vi "spl.vi"() -> ()   [LabVIEW 2017]
doc: "Performs limit testing on unevenly sampled data. You might have unevenly sampled data in some applications, such as data sampled on a logarithmic scale.\n\nThis example uses the Limit Specification for Unevenly Sampled Data subVI. If you do not wire the dx and the x0 inputs, this VI accepts an array of X axis values at which your signal is sampled. It creates the limit at these X values. The example then uses the Limit Testing VI to compare the signal with the limits."
uses:
  <vilib>/measure/mamon.llb/Limit Testing Time.vi
  <vilib>/measure/NI_MAPro.lvlib
panel:
  in  "声压级":dbl[](array[numeric])=[82.29, 84.67, 86.31, 87.22, 86.54, 84.99, 83.09, 82.19, 82.2, 83.13, 84.47, 86.53, 88.83, 91.58, 93.49, 94.45, 94.45, 93.83, 93.46, 94.46, 97.18, 99.83, 101.28, 102.07, 102.67, 103.01, 102.91, 102.6, 101.82, 100.98, 99.07, 98.85, 101.46, 101.31, 99.62, 101.88, 104.09, 102.62, 103.66, 103.86, 104.63, 105.12, 105.52, 103.79, 103.37, 103.81, 105.35, 105.82, 105.16, 103.88, 102.23, 101.82, 102.49, 102.97, 100.5, 101.51, 101.54, 101.41, 101.61, 101.8, 102.8]
  in  "频率":dbl[](array[numeric])=[204.0, 216.0, 227.0, 241.0, 255.0, 270.0, 285.0, 302.0, 319.0, 338.0, 357.0, 378.0, 399.0, 422.0, 446.0, 472.0, 499.0, 528.0, 558.0, 590.0, 623.0, 659.0, 697.0, 736.0, 778.0, 823.0, 870.0, 919.0, 972.0, 1025.0, 1086.0, 1149.0, 1214.0, 1288.0, 1358.0, 1435.0, 1517.0, 1606.0, 1695.0, 1796.0, 1898.0, 2005.0, 2130.0, 2242.0, 2371.0, 2508.0, 2649.0, 2802.0, 2961.0, 3126.0, 3315.0, 3500.0, 3695.0, 3911.0, 4136.0, 4372.0, 4630.0, 4889.0, 5169.0, 5461.0, 5783.0]
  out "test passed?":bool=TRUE
  out "Limit Test":T1(graph)=[{"X Values for Signal"=[204.0, 216.0, 227.0, 241.0, 255.0, 270.0, 285.0, 302.0, 319.0, 338.0, 357.0, 378.0, 399.0, 422.0, 446.0, 472.0, 499.0, 528.0, 558.0, 590.0, 623.0, 659.0, 697.0, 736.0, 778.0, 823.0, 870.0, 919.0, 972.0, 1025.0, 1086.0, 1149.0, 1214.0, 1288.0, 1358.0, 1435.0, 1517.0, 1606.0, 1695.0, 1796.0, 1898.0, 2005.0, 2130.0, 2242.0, 2371.0, 2508.0, 2649.0, 2802.0, 2961.0, 3126.0, 3315.0, 3500.0, 3695.0, 3911.0, 4136.0, 4372.0, 4630.0, 4889.0, 5169.0, 5461.0, 5783.0], "Y"=[82.29, 84.67, 86.31, 87.22, 86.54, 84.99, 83.09, 82.19, 82.2, 83.13, 84.47, 86.53, 88.83, 91.58, 93.49, 94.45, 94.45, 93.83, 93.46, 94.46, 97.18, 99.83, 101.28, 102.07, 102.67, 103.01, 102.91, 102.6, 101.82, 100.98, 99.07, 98.85, 101.46, 101.31, 99.62, 101.88, 104.09, 102.62, 103.66, 103.86, 104.63, 105.12, 105.52, 103.79, 103.37, 103.81, 105.35, 105.82, 105.16, 103.88, 102.23, 101.82, 102.49, 102.97, 100.5, 101.51, 101.54, 101.41, 101.61, 101.8, 102.8]}, {"X Values for Signal"=[204.0, 216.0, 227.0, 241.0, 255.0, 270.0, 285.0, 302.0, 319.0, 338.0, 357.0, 378.0, 399.0, 422.0, 446.0, 472.0, 499.0, 528.0, 558.0, 590.0, 623.0, 659.0, 697.0, 736.0, 778.0, 823.0, 870.0, 919.0, 972.0, 1025.0, 1086.0, 1149.0, 1214.0, 1288.0, 1358.0, 1435.0, 1517.0, 1606.0, 1695.0, 1796.0, 1898.0, 2005.0, 2130.0, 2242.0, 2371.0, 2508.0, 2649.0, 2802.0, 2961.0, 3126.0, 3315.0, 3500.0, 3695.0, 3911.0, 4136.0, 4372.0, 4630.0, 4889.0, 5169.0, 5461.0, 5783.0], "Y"=[nan, nan, nan, nan, nan, nan, nan, nan, nan, nan, nan, nan, nan, nan, nan, nan, nan, nan, nan, nan, nan, nan, nan, nan, nan, nan, nan, nan, nan, nan, nan, nan, nan, nan, nan, nan, nan, nan, nan, nan, nan, nan, nan, nan, nan, nan, nan, nan, nan, nan, nan, nan, nan, nan, nan, nan, nan, nan, nan, nan, nan]}, {"X Values for Signal"=[204.0, 216.0, 227.0, 241.0, 255.0, 270.0, 285.0, 302.0, 319.0, 338.0, 357.0, 378.0, 399.0, 422.0, 446.0, 472.0, 499.0, 528.0, 558.0, 590.0, 623.0, 659.0, 697.0, 736.0, 778.0, 823.0, 870.0, 919.0, 972.0, 1025.0, 1086.0, 1149.0, 1214.0, 1288.0, 1358.0, 1435.0, 1517.0, 1606.0, 1695.0, 1796.0, 1898.0, 2005.0, 2130.0, 2242.0, 2371.0, 2508.0, 2649.0, 2802.0, 2961.0, 3126.0, 3315.0, 3500.0, 3695.0, 3911.0, 4136.0, 4372.0, 4630.0, 4889.0, 5169.0, 5461.0, 5783.0], "Y"=[nan, nan, nan, nan, nan, nan, nan, 88.2, 89.9, 91.8, 93.7, 95.8, 97.9, 98.495, 99.035, 99.62, 100.2275, 100.88, 101.555, 102.275, 103.0175, 103.8275, 104.6825, 105.56, 106.505, 106.885, 106.65, 106.405, 106.14, 105.875, 105.57, 105.255, 105.0525, 105.33, 105.5925, 105.88125, 106.18875, 106.5225, 106.85625, 107.235, 107.6175, 108.0, 108.0, 108.0, 108.0, 108.0, 108.0, 108.0, 108.0, 108.0, 108.0, 108.0, 107.7075, 107.3835, 107.046, 106.69200000000001, 106.305, 105.9165, 105.4965, 105.0585, nan]}, {"X Values for Signal"=[204.0, 216.0, 227.0, 241.0, 255.0, 270.0, 285.0, 302.0, 319.0, 338.0, 357.0, 378.0, 399.0, 422.0, 446.0, 472.0, 499.0, 528.0, 558.0, 590.0, 623.0, 659.0, 697.0, 736.0, 778.0, 823.0, 870.0, 919.0, 972.0, 1025.0, 1086.0, 1149.0, 1214.0, 1288.0, 1358.0, 1435.0, 1517.0, 1606.0, 1695.0, 1796.0, 1898.0, 2005.0, 2130.0, 2242.0, 2371.0, 2508.0, 2649.0, 2802.0, 2961.0, 3126.0, 3315.0, 3500.0, 3695.0, 3911.0, 4136.0, 4372.0, 4630.0, 4889.0, 5169.0, 5461.0, 5783.0], "Y"=[nan, nan, nan, nan, nan, nan, nan, 79.04, 79.38, 79.76, 80.14, 80.56, 80.98, 81.99, 83.07, 84.24, 85.455, 86.76, 88.11, 89.55, 91.035, 92.655, 94.36500000000001, 96.12, 98.00999999999999, 98.9425, 98.825, 98.7025, 98.57, 98.4375, 98.285, 98.1275, 98.035, 98.22, 98.395, 98.5875, 98.7925, 99.015, 99.2375, 99.49, 99.745, 99.99333333333334, 99.82666666666667, 99.67733333333334, 99.50533333333334, 99.32266666666666, 99.13466666666666, 98.93066666666667, 98.71866666666666, 98.49866666666667, 98.24666666666667, 98.0, 98.0, 98.0, 98.0, 98.0, 98.0, 98.0, 98.0, 98.0, nan]}]
  # "Overview: This example shows how to run a limit test on unevenly sampled data.\nRequirements: LabVIEW Full Development System\nInstructions: \n1. Run the VI.  \n2. Change the Y values for Signal to contain values above the Upper Limit or below the Lower Limit and run the VI again. The limit test should fail."
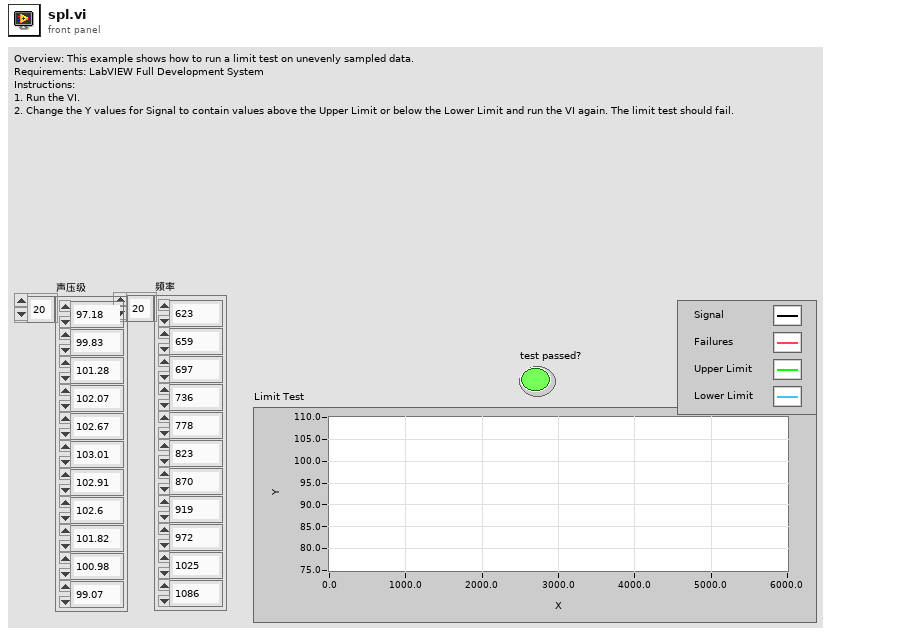
[diagram p1: front panel]
types:
  T1 = cluster{"X Values for Signal":dbl[], "Y":dbl[]}[]
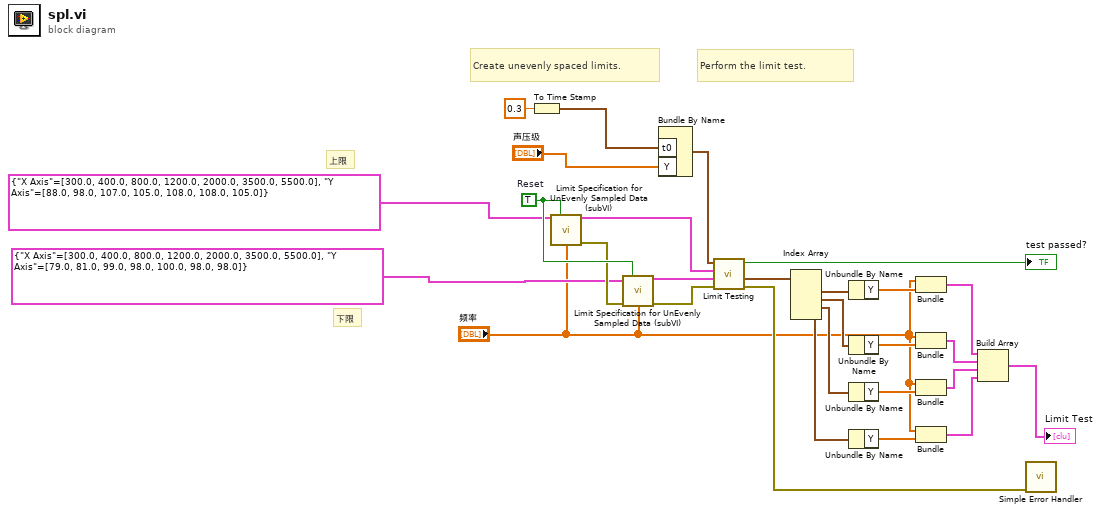
[diagram p0: block diagram]
diagram:
  w8 = TRUE  # Reset
  # "下限"
  # "上限"
  # "Perform the limit test."
  # "Create unevenly spaced limits."
  n1 = To Time Stamp(1:0.3) -> (0:w12:timestamp)
  n2 = call "Limit Specification for UnEvenly Sampled Data (subVI).vi"("Specification Cluster"=cluster{"X Axis":dbl[], "Y Axis":dbl[]} {"X Axis"=[300.0, 400.0, 800.0, 1200.0, 2000.0, 3500.0, 5500.0], "Y Axis"=[88.0, 98.0, 107.0, 105.0, 108.0, 108.0, 105.0]}, "reset"=w8, "X Values for Signal"="频率") -> ("Limit"=w14:cluster{"x0":dbl, "dx":dbl, "Y":dbl[]}, "error out"=w6:errorcluster)  [unwired: 11 in]
  n3 = call "Limit Specification for UnEvenly Sampled Data (subVI).vi"("Specification Cluster"=cluster{"X Axis":dbl[], "Y Axis":dbl[]} {"X Axis"=[300.0, 400.0, 800.0, 1200.0, 2000.0, 3500.0, 5500.0], "Y Axis"=[79.0, 81.0, 99.0, 98.0, 100.0, 98.0, 98.0]}, "reset"=w8, "error in (no error)"=w6, "X Values for Signal"="频率") -> ("Limit"=w13:cluster{"x0":dbl, "dx":dbl, "Y":dbl[]}, "error out"=w5:errorcluster)  [unwired: 10 in]
  n4 = Bundle By Name("t0"=w12, "Y"="声压级") -> (w24:waveform(dbl))  [unwired: 1 in]
  n5 = call-poly <vilib>:"Limit Testing.vi"("error in (no error)"=w5, "lower limit"=w13, "upper limit"=w14, "signal in"=w24) -> ("error out"=w7:errorcluster, "output values"=w23:waveform(dbl)[], "test passed?"=→"test passed?":bool)  [unwired: 2 in, 3 out]
  n6 = Index Array(array=w23) -> (element #1=w22:waveform(dbl), element #2=w11:waveform(dbl), element #3=w10:waveform(dbl), element #4=w9:waveform(dbl))  [unwired: 4 in]
  n7 = Unbundle By Name(w22) -> ("Y"=w21:dbl[])
  n8 = Unbundle By Name(w11) -> ("Y"=w20:dbl[])
  n9 = Unbundle By Name(w10) -> ("Y"=w19:dbl[])
  n10 = Unbundle By Name(w9) -> ("Y"=w18:dbl[])
  n11 = Bundle("频率"="频率", "Y"=w21) -> (w27:cluster{"频率":dbl[], "Y":dbl[]})  [unwired: 1 in]
  n12 = Bundle("频率"="频率", "Y"=w20) -> (w26:cluster{"频率":dbl[], "Y":dbl[]})  [unwired: 1 in]
  n13 = Bundle("频率"="频率", "Y"=w19) -> (w25:cluster{"频率":dbl[], "Y":dbl[]})  [unwired: 1 in]
  n14 = Bundle("频率"="频率", "Y"=w18) -> (w16:cluster{"频率":dbl[], "Y":dbl[]})  [unwired: 1 in]
  n15 = Build Array(w27, w26, w25, w16) -> (→"Limit Test":cluster{"频率":dbl[], "Y":dbl[]}[])
  n16 = call <vilib>:"Simple Error Handler.vi"("error in (no error)"=w7) -> ()  [unwired: 4 in, 5 out]
